vi "LDA_U16_data_header.vi"() -> (0 "Output string":string)   [LabVIEW 2011]
uses:
  Globals/Meas_global.vi
  Globals/LDA_meas_global_1.vi
  Globals/LDA_meas_global_2.vi
panel:
  out "length":i32
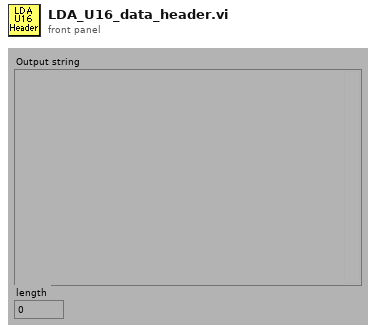
[diagram p1: front panel]
types:
  T1 = typedef "LDA_Setup.ctl" = cluster{"dimensions":enum16{"1D", "2D"}, "Analogue Freq Multiplier":dbl}
  T2 = typedef "BSA_Type.ctl" = enum16{"57N11", "BSA F60"}
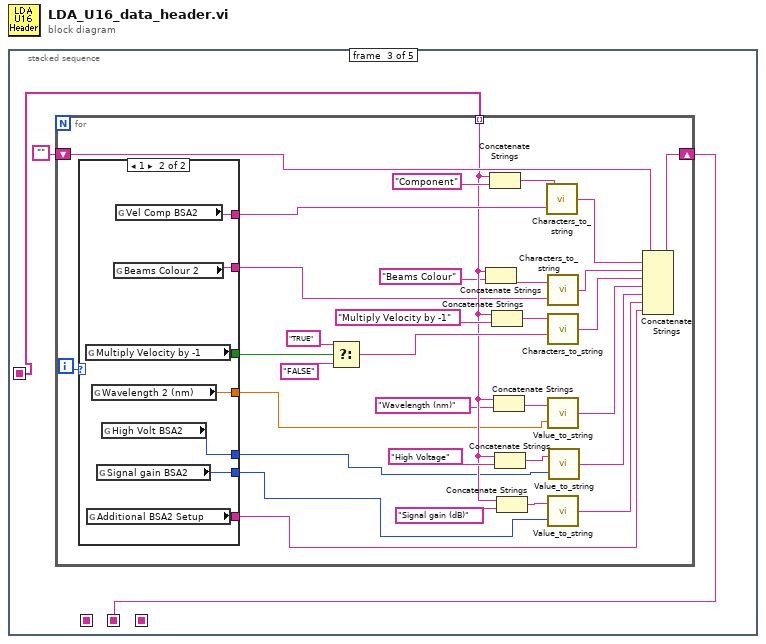
[diagram p0: block diagram]
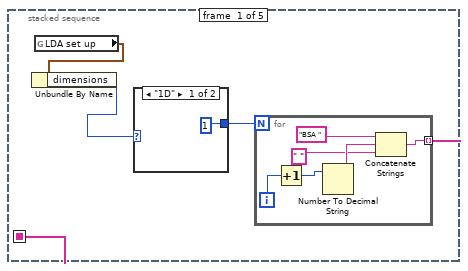
[diagram p2: hidden frame]
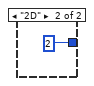
[diagram p3: hidden frame]
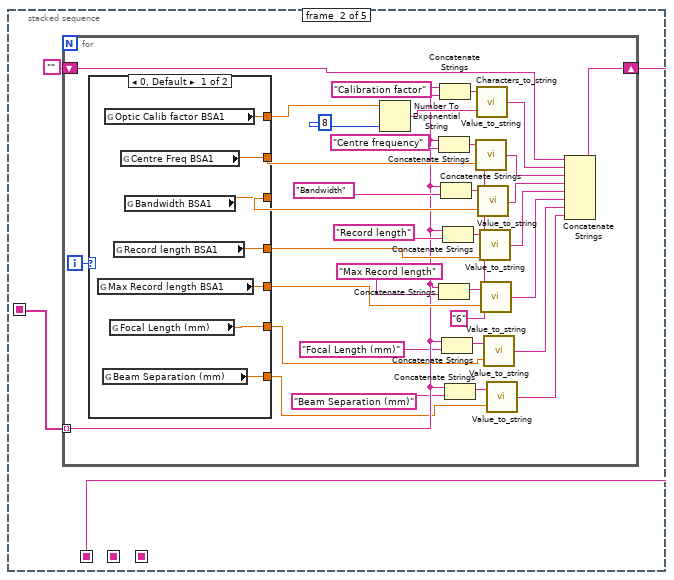
[diagram p4: hidden frame]
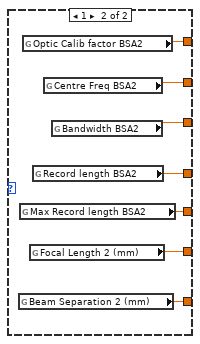
[diagram p5: hidden frame]
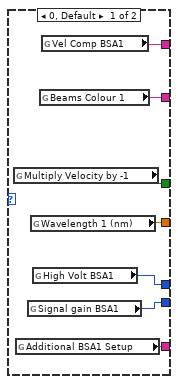
[diagram p6: hidden frame]
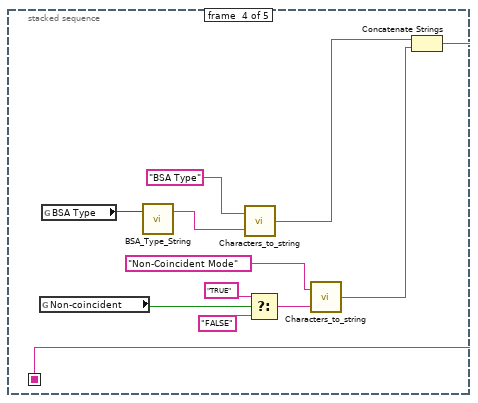
[diagram p7: hidden frame]
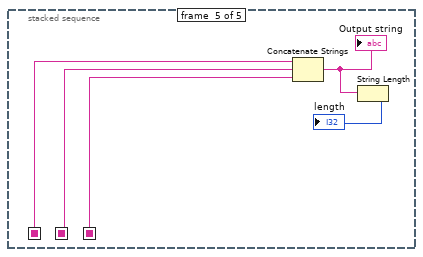
[diagram p8: hidden frame]
diagram:
  n1 = stacked-sequence {
    seq-local: [_ w14 _ _ _] -> [_ _ _ _ w129]
    seq-local: [_ _ w66 _ _] -> [_ _ _ _ w128]
    seq-local: [w4 _ _ _ _] -> [_ w13 w65 _ _]
    seq-local: [_ _ _ w124 _] -> [_ _ _ _ w125]
    frame #0 {
      n2 = global read "Meas_global.vi" "LDA set up"() -> (w2:T1)
      n3 = Unbundle By Name(w2) -> ("dimensions"=w1:enum16{"1D", "2D"})
      n4 = case shown="\"1D\"" w1 {
        tunnel: [1 2] -> w3
        frame "1D" {
        }
        frame "2D" {
        }
      }
      n5 = for {
        N: w3 -> [_]
        tunnel: [w9] -> w4 mode=indexing
        i -> [w7]
        n6 = Increment(x=w7) -> (x+1=w10:i32)
        n7 = Number To Decimal String(number=w10) -> (decimal integer string=w12:string)  [unwired: 1 out]
        n8 = Concatenate Strings("BSA ", w12, " ") -> (w9:string)
      }
    }
    frame #1 {
      n9 = for {
        shift-right: [w48] -> w14
        shift-left: "" -> [w49]
        tunnel: w13 -> [w22] mode=indexing
        i -> [w50]
        w28 = "6" ("precision")
        n10 = case shown="0, Default" w50 {
          tunnel: [w57 w61] -> w26
          tunnel: [w56 w62] -> w41
          tunnel: [w55 w63] -> w42
          tunnel: [w54 w64] -> w43
          tunnel: [w53 w60] -> w30
          tunnel: [w52 w58] -> w17
          tunnel: [w51 w59] -> w16
          frame 0, Default {
            n11 = global read "LDA_meas_global_1.vi" "Max Record length BSA1"() -> (w53:dbl)
            n12 = global read "LDA_meas_global_1.vi" "Beam Separation (mm)"() -> (w51:dbl)
            n13 = global read "LDA_meas_global_1.vi" "Optic Calib factor BSA1"() -> (w57:dbl)
            n14 = global read "LDA_meas_global_1.vi" "Focal Length (mm)"() -> (w52:dbl)
            n15 = global read "LDA_meas_global_1.vi" "Record length BSA1"() -> (w54:dbl)
            n16 = global read "LDA_meas_global_1.vi" "Centre Freq BSA1"() -> (w56:dbl)
            n17 = global read "LDA_meas_global_1.vi" "Bandwidth BSA1"() -> (w55:dbl)
          }
          frame 1 {
            n18 = global read "LDA_meas_global_2.vi" "Beam Separation 2 (mm)"() -> (w59:dbl)
            n19 = global read "LDA_meas_global_2.vi" "Max Record length BSA2"() -> (w60:dbl)
            n20 = global read "LDA_meas_global_2.vi" "Optic Calib factor BSA2"() -> (w61:dbl)
            n21 = global read "LDA_meas_global_2.vi" "Focal Length 2 (mm)"() -> (w58:dbl)
            n22 = global read "LDA_meas_global_2.vi" "Record length BSA2"() -> (w64:dbl)
            n23 = global read "LDA_meas_global_2.vi" "Centre Freq BSA2"() -> (w62:dbl)
            n24 = global read "LDA_meas_global_2.vi" "Bandwidth BSA2"() -> (w63:dbl)
          }
        }
        n25 = Number To Exponential String(number=w26, precision (6)=i16 8) -> (E-format string=w25:string)  [unwired: 2 out]
        n26 = Concatenate Strings(w22, "Centre frequency") -> (w46:string)
        n27 = Concatenate Strings(w22, "Max Record length") -> (w31:string)
        n28 = Concatenate Strings(w22, "Calibration factor") -> (w47:string)
        n29 = Concatenate Strings(w22, "Bandwidth") -> (w45:string)
        n30 = Concatenate Strings(w22, "Focal Length (mm)" ("Label for characters")) -> (w24:string)
        n31 = Concatenate Strings(w22, "Record length") -> (w44:string)
        n32 = Concatenate Strings(w22, "Beam Separation (mm)" ("Label for characters")) -> (w23:string)
        n33 = call "Value_to_string.vi"("precision"=w28, "Value"=w41, "Label for value"=w46) -> ("Output string"=w39:string)
        n34 = call "Characters_to_string.vi"("Characters to write"=w25, "Label for characters"=w47) -> ("Output string"=w40:string)
        n35 = call "Value_to_string.vi"("precision"=w28, "Value"=w42, "Label for value"=w45) -> ("Output string"=w38:string)
        n36 = call "Value_to_string.vi"("precision"=w28, "Value"=w43, "Label for value"=w44) -> ("Output string"=w33:string)
        n37 = call "Value_to_string.vi"("precision"=w28, "Value"=w30, "Label for value"=w31) -> ("Output string"=w29:string)
        n38 = call "Value_to_string.vi"("Value"=w17, "Label for value"=w24) -> ("Output string"=w19:string)  [unwired: 1 in]
        n39 = call "Value_to_string.vi"("Value"=w16, "Label for value"=w23) -> ("Output string"=w18:string)  [unwired: 1 in]
        n40 = Concatenate Strings(w49, w40, w39, w38, w33, w29, w19, w18) -> (w48:string)
      }
    }
    frame #2 {
      n41 = for {
        shift-right: [w97] -> w66
        shift-left: "" -> [w98]
        tunnel: w65 -> [w78] mode=indexing
        i -> [w99]
        n42 = case shown="1" w99 {
          tunnel: [w106 w113] -> w68
          tunnel: [w105 w112] -> w93
          tunnel: [w104 w111] -> w90
          tunnel: [w102 w110] -> w72
          tunnel: [w103 w109] -> w71
          tunnel: [w101 w108] -> w70
          tunnel: [w100 w107] -> w69
          frame 0, Default {
            n43 = global read "LDA_meas_global_1.vi" "Multiply Velocity by -1"() -> (w104:bool)
            n44 = global read "LDA_meas_global_1.vi" "Additional BSA1 Setup"() -> (w101:string)
            n45 = global read "LDA_meas_global_1.vi" "Signal gain BSA1"() -> (w102:i16)
            n46 = global read "LDA_meas_global_1.vi" "Wavelength 1 (nm)"() -> (w100:dbl)
            n47 = global read "LDA_meas_global_1.vi" "High Volt BSA1"() -> (w103:i16)
            n48 = global read "LDA_meas_global_1.vi" "Beams Colour 1"() -> (w106:string)
            n49 = global read "LDA_meas_global_1.vi" "Vel Comp BSA1"() -> (w105:string)
          }
          frame 1 {
            n50 = global read "LDA_meas_global_2.vi" "Multiply Velocity by -1"() -> (w111:bool)
            n51 = global read "LDA_meas_global_2.vi" "Additional BSA2 Setup"() -> (w108:string)
            n52 = global read "LDA_meas_global_2.vi" "Wavelength 2 (nm)"() -> (w107:dbl)
            n53 = global read "LDA_meas_global_2.vi" "Signal gain BSA2"() -> (w110:i16)
            n54 = global read "LDA_meas_global_2.vi" "High Volt BSA2"() -> (w109:i16)
            n55 = global read "LDA_meas_global_2.vi" "Beams Colour 2"() -> (w113:string)
            n56 = global read "LDA_meas_global_2.vi" "Vel Comp BSA2"() -> (w112:string)
          }
        }
        n57 = Select(t="TRUE" ("y"), s=w90, f="FALSE" ("y")) -> (s? t:f=w87:string)
        n58 = Concatenate Strings(w78, "Beams Colour" ("string")) -> (w84:string)
        n59 = Concatenate Strings(w78, "Component") -> (w96:string)
        n60 = Concatenate Strings(w78, "Multiply Velocity by -1") -> (w91:string)
        n61 = Concatenate Strings(w78, "Wavelength (nm)") -> (w83:string)
        n62 = Concatenate Strings(w78, "High Voltage") -> (w82:string)
        n63 = Concatenate Strings(w78, "Signal gain (dB)") -> (w81:string)
        n64 = call "Characters_to_string.vi"("Characters to write"=w93, "Label for characters"=w96) -> ("Output string"=w95:string)
        n65 = call "Characters_to_string.vi"("Characters to write"=w68, "Label for characters"=w84) -> ("Output string"=w85:string)
        n66 = call "Characters_to_string.vi"("Characters to write"=w87, "Label for characters"=w91) -> ("Output string"=w86:string)
        n67 = call "Value_to_string.vi"("Value"=w69, "Label for value"=w83) -> ("Output string"=w75:string)  [unwired: 1 in]
        n68 = call "Value_to_string.vi"("Value"=w72, "Label for value"=w81) -> ("Output string"=w77:string)  [unwired: 1 in]
        n69 = call "Value_to_string.vi"("Value"=w71, "Label for value"=w82) -> ("Output string"=w76:string)  [unwired: 1 in]
        n70 = Concatenate Strings(w98, w95, w85, w86, w75, w76, w77, w70) -> (w97:string)
      }
    }
    frame #3 {
      n71 = global read "LDA_meas_global_1.vi" "Non-coincident"() -> (w117:bool)
      n72 = global read "LDA_meas_global_1.vi" "BSA Type"() -> (w123:T2)
      n73 = call "BSA_Type_String.vi"("BSA Type"=w123) -> ("BSA String Out"=w122:string)  [unwired: 1 in, 1 out]
      n74 = call "Characters_to_string.vi"("Characters to write"=w122, "Label for characters"="BSA Type") -> ("Output string"=w121:string)
      n75 = Select(t="TRUE" ("y"), s=w117, f="FALSE" ("y")) -> (s? t:f=w116:string)
      n76 = call "Characters_to_string.vi"("Characters to write"=w116, "Label for characters"="Non-Coincident Mode") -> ("Output string"=w115:string)
      n77 = Concatenate Strings(w121, w115) -> (w124:string)
    }
    frame #4 {
      n78 = Concatenate Strings(w129, w128, w125) -> (w126:string)
      "Output string" <- w126
      n79 = String Length(string=w126) -> (length=→"length":i32)
    }
  }
